vi "Configure Measurement.vi"(0 "VISA resource name":refnum<visa-resource-name>, 5 "Window Type (1: KBessel)":u16(ring)=1 items=["Rectangular", "KBessel"], 7 "Relative Trigger Samples (0)":i32, 9 "Sample Spacing (25 us)":dbl=2.5e-05 format="%^.2g", 11 "error in (no error)":errorcluster) -> (4 "VISA resource name out":refnum<visa-resource-name>, 15 "error out":errorcluster)   [LabVIEW 2020, in "Agilent 681x Series.lvlib"]
doc: "Configures the measurement window, sweep points and sample spacing."
uses:
  <instrlib>/Agilent 681x Series/Agilent 681x Series.lvlib
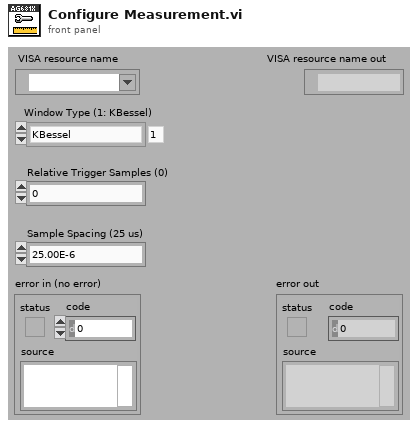
[diagram p1: front panel]
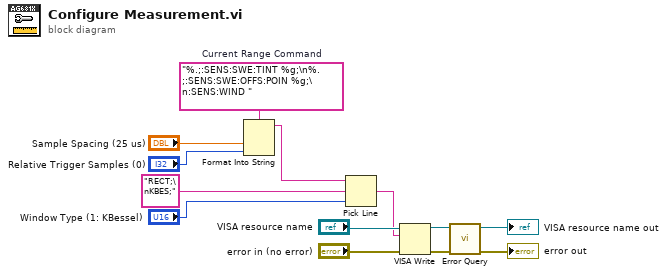
[diagram p0: block diagram]
diagram:
  w9 = "%.;:SENS:SWE:TINT %g;\n%.;:SENS:SWE:OFFS:POIN %g;\n:SENS:WIND "  # Current Range Command
  n1 = Format Into String(format string=w9, "Sample Spacing (25 us)", "Relative Trigger Samples (0)") -> (resulting string=w4:string)  [unwired: 2 in, 1 out]
  n2 = Pick Line(string ("")=w4, multi-line string="RECT;\nKBES;", line index="Window Type (1: KBessel)") -> (output string=w1:string)
  n3 = VISA Write(VISA resource name="VISA resource name", write buffer=w1, error in (no error)="error in (no error)") -> (VISA resource name out=w11:refnum<visa-resource-name>, error out=w10:errorcluster)  [unwired: 1 out]
  n4 = call <instrlib>:"Error Query.vi"("error in (no error)"=w10, "VISA resource name"=w11) -> ("error out"=→"error out":errorcluster, "VISA resource name out"=→"VISA resource name out":refnum<visa-resource-name>)  [unwired: 6 in, 2 out]
